vi "Set Magnet.vi"(4 "Mode":T2, 6 "Axis":T1, 8 "error in (no error)":errorcluster, 9 "Target Rate (T/min)":dbl, 10 "Target Field (T)":dbl, 11 "instrument.PPMS in":refnum<class "instrument.PPMS1.lvclass">) -> (0 "error out":errorcluster, 3 "instrument.PPMS out":refnum<class "instrument.PPMS1.lvclass">)   [LabVIEW 2019, in "instrument.PPMS1.lvclass"]
uses:
  instrument.PPMS1.lvclass
  <userlib>/LevyLab/Levylab Instruments/Instrument Types/Cryostat/Typedefs/Magnet Mode--Enum.ctl
  <userlib>/LevyLab/Levylab Instruments/Instrument Types/Cryostat/Typedefs/Magnet Axis--Enum.ctl
  Typedefs/PPMS1.Commands-enum.ctl
  <userlib>/LevyLab/Levylab Instruments/Instrument Types/Cryostat/Typedefs/Set Magnet--cluster.ctl
  43145f45-1774-454b-b412-69884133393d.vi
  43145f45-1774-454b-b412-69884133393d.vi/1c80e656-119e-415d-885e-a6d1bc4fb436.vi
  <userlib>/LevyLab/Levylab Instruments/SMOs/RemoteControl/API/Remote Client.vi
  <userlib>/LevyLab/Levylab Instruments/Instrument Types/Cryostat/Instrument.Cryostat.lvclass
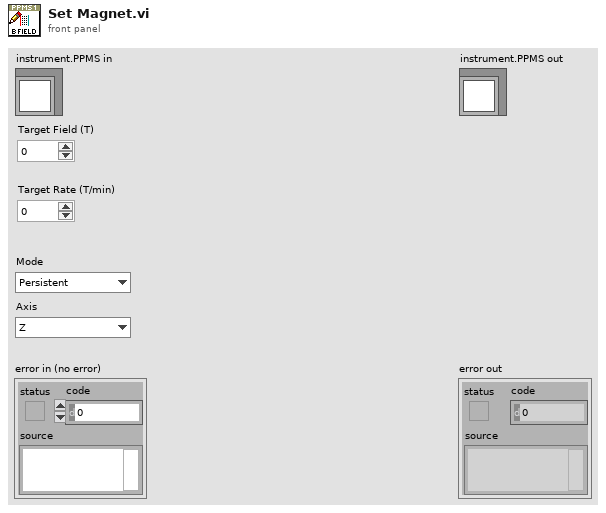
[diagram p1: front panel]
types:
  T1 = typedef "Instrument.Cryostat.lvclass/Magnet Axis--Enum.ctl" = enum16{"Z", "X", "Y"}
  T2 = typedef "Instrument.Cryostat.lvclass/Magnet Mode--Enum.ctl" = enum16{"Persistent", "Driven"}
  T3 = typedef "Instrument.Cryostat.lvclass/Set Magnet--cluster.ctl" = cluster{"Field (T)":dbl, "Rate (T/min)":dbl, "Axis":T1, "Mode":T2}
  T4 = typedef "instrument.PPMS1.lvclass/PPMS1.Commands-enum.ctl" = enum16{"Get Magnet Field", "Get Helium Level", "Get Temperature", "Set Magnet Field", "Set Temperature", "getAll"}
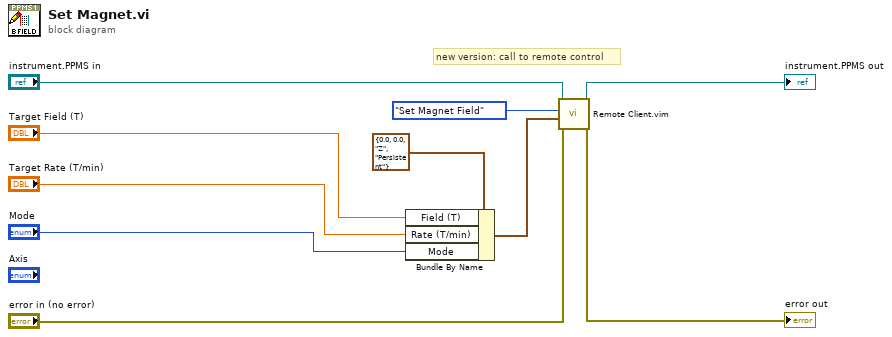
[diagram p0: block diagram]
diagram:
  # "new version: call to remote control"
  n1 = Bundle By Name(cluster=T3 {"Field (T)"=0.0, "Rate (T/min)"=0.0, "Axis"=enum."Z", "Mode"=enum."Persistent"} ("Set Magnet Field"), "Field (T)"="Target Field (T)", "Rate (T/min)"="Target Rate (T/min)", "Mode"="Mode") -> (w4:T3)
  n2 = call "Remote Client.vim"("error in (no error)"="error in (no error)", "Data"=w4, "Command"=PPMS1.Commands-enum."Set Magnet Field", "Instrument in"="instrument.PPMS in") -> ("error out"=→"error out":errorcluster, "Instrument out"=→"instrument.PPMS out":refnum<class "instrument.PPMS1.lvclass">)  [unwired: 4 in, 2 out]
